vi "Read Device Identification.vi"(8 "error in (no error)":errorcluster, 9 "read device ID code":T1, 10 "object ID":u8, 11 "Modbus master in":refnum<class "Network Master.lvclass">) -> (0 "error out":errorcluster, 2 "objects":cluster{"object ID":u8, "value":string}[](array[cluster]) {"object ID" format="%x"}, 3 "Modbus master out":refnum<class "Network Master.lvclass">)   [LabVIEW 2021, in "Network Master.lvclass"]
doc: "Returns the device identification of a Modbus slave. Device identification consists of data elements called objects. Each object has an identification number and stores Modbus slave information."
uses:
  Network Master.lvclass
  D:/my_projects/projects/Algorithms/Labview/21/Modbus_v121c/Network Protocol/Network Protocol.lvclass
  Master Function Definition/Read Device ID code.ctl
  Data Model/Identification Parameters.ctl
  Modbus Data Unit/Modbus Data Unit.lvclass/Modbus Data Unit.ctl
  Network Protocol.lvclass/Network Protocol.ctl
  Network Master.lvclass/Network Master.ctl
  Modbus Data Unit/Construct PDU.vi
  Read Transmission Data Unit.vi
  Master Function Definition/Convert to String.vi
  Master Function Definition/Function code mismatch error.vi
  Data Model/Error Generator.vi
  Modbus Data Unit/Deconstruct PDU.vi
  Modbus Data Unit/Modbus Data Unit.lvclass
  Transmission Data Unit/Transmission Data Unit.lvclass
  Master Function Definition/Master Function Definition.lvclass
  Data Model/Device Data Model.lvclass
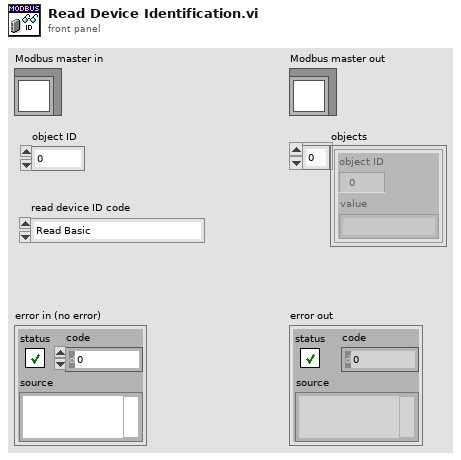
[diagram p1: front panel]
types:
  T1 = typedef "Device Data Model.lvclass/Read Device ID code.ctl" = enum8{"Read Basic", "Read Regular", "Read Extended", "Read Specific"}
  T2 = typedef "Device Data Model.lvclass/Identification Parameters.ctl" = cluster{"Object ID":u8, "Value":string}
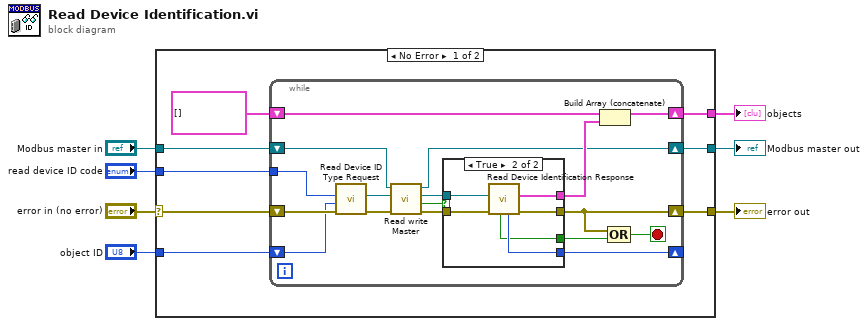
[diagram p0: block diagram]
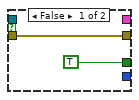
[diagram p2: hidden frame]
diagram:
  n1 = case shown="No Error" "error in (no error)" {
    selector: "error in (no error)" -> [w8 w42]
    tunnel: "Modbus master in" -> [w9 w41]
    tunnel: [w10 w41] -> w5
    tunnel: [w11 w42] -> w4
    tunnel: "read device ID code" -> [w15 _]
    tunnel: "object ID" -> [w14 _]
    tunnel: [w13 _] -> w2
    frame No Error {
      n2 = while {
        tunnel: w15 -> [w31]
        shift-right: [w28] -> w11
        shift-left: w8 -> [w32]
        shift-right: [w27] -> w13
        shift-left: T2[] [] -> [w26]
        shift-right: [w25] -> _
        shift-left: w14 -> [w30]
        shift-right: [w16] -> w10
        shift-left: w9 -> [w17]
        stop <- w29 stop-if-true
        n3 = call "Read Device ID Type Request.vi"("error in"=w32, "Object ID"=w30, "Read Device ID Code"=w31) -> ("error out"=w21:errorcluster, "modbus data unit out"=w18:refnum<class "Modbus Data Unit.lvclass">)  [unwired: 7 in]
        n4 = call "Read write Master.vi"("error in (no error)"=w21, "Modbus data unit in"=w18, "Modbus master in"=w17) -> ("error out"=w22:errorcluster, "PDU valid?"=w20:bool, "Modbus data unit out"=w19:refnum<class "Modbus Data Unit.lvclass">, "Modbus master out"=w16:refnum<class "Network Master.lvclass">)  [unwired: 5 in]
        n5 = case shown="True" w20 {
          tunnel: [w34 w40] -> w28
          tunnel: [_ w39] -> w25
          tunnel: [TRUE ("done?") w38] -> w24
          tunnel: [_ w37] -> w23
          tunnel: w22 -> [w34 w36]
          tunnel: w19 -> [_ w35]
          frame False {
          }
          frame True {
            n6 = call "Read Device Identification Response.vi"("error in"=w36, "modbus data unit in"=w35) -> ("error out"=w40:errorcluster, "Objects"=w37:T2[], "Next Object ID"=w39:u8, "done?"=w38:bool)  [unwired: 5 in, 1 out]
          }
        }
        n7 = Build Array (concatenate)(w26, w23) -> (w27:T2[])
        n8 = Compound Arithmetic op=OR(w28, w24) -> (w29:bool)
      }
    }
    frame Error {
    }
  }
  "error out" <- w4
  "Modbus master out" <- w5
  "objects" <- w2
